vi "Request Identities.vi"(8 "Error In":errorcluster, 11 "Agent In":refnum<class "Agent.lvclass">) -> (0 "Error Out":errorcluster, 3 "Agent Out":refnum<class "Agent.lvclass">)   [LabVIEW 2018, in "Toolkit.lvlib" / "Agent.lvclass"]
doc: "Obtain a list of identities that are available from a running instance of a SSH agent application. The identities are returned from the SSH agent application as a linked list internal to the libssh2 library. This VI must be called before transversal of the linked list with the First and Next VIs."
uses:
  Agent.lvclass
  Agent.lvclass/Agent.ctl
  Session/Session.lvclass/Session.ctl
  SSH/SSH.lvclass/SSH.ctl
  Toolkit.lvlib
  Session/Session.lvclass
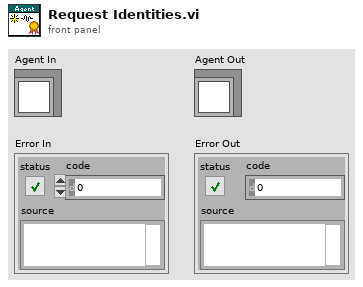
[diagram p1: front panel]
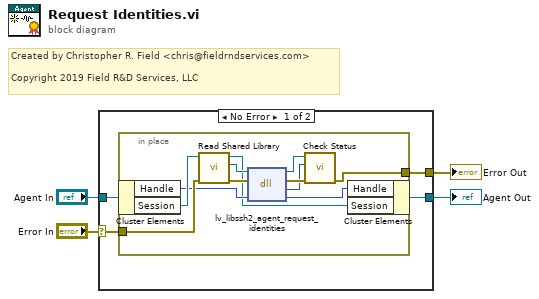
[diagram p0: block diagram]
diagram:
  # "Created by Christopher R. Field <chris@fieldrndservices.com>\n\nCopyright 2019 Field R&D Services, LLC"
  n1 = case shown="No Error" "Error In" {
    selector: "Error In" -> [w7 w21]
    tunnel: [w8 w21] -> w3
    tunnel: "Agent In" -> [w6 w20]
    tunnel: [w5 w20] -> w1
    frame No Error {
      n2 = in-place {
        in-place-border: [w16] -> w8
        in-place-border: w7 -> [w11]
        n3 = in-place-cluster #1(w6) -> ("Handle"=w10:u64, "Session"=w14:refnum<class "Session.lvclass">)
        n4 = call "Read Shared Library.vi"("Error In"=w11, "Session In"=w14) -> ("Erorr Out"=w12:errorcluster, "libssh2lv Shared Library"=w13:path, "Session Out"=w9:refnum<class "Session.lvclass">)  [unwired: 7 in]
        n5 = dll-call lib="libssh2lv.*" fn="lv_libssh2_agent_request_identities"(path in=w13, error in=w12, "handle"=w10) -> (path out=w17:path, error out=w18:errorcluster, "result"=w15:i32, "handle"=w19:u64)  [unwired: 1 in]
        n6 = call "Check Status.vi"("Error In"=w18, "Status"=w15, "lv-libssh2 Shared Library In"=w17) -> ("Error Out"=w16:errorcluster)  [unwired: 7 in, 1 out]
        n7 = in-place-cluster #1("Handle"=w19, "Session"=w9) -> (w5:refnum<class "Agent.lvclass">)
      }
    }
    frame Error {
    }
  }
  "Error Out" <- w3
  "Agent Out" <- w1
